vi "Initialize.vi"(8 "error in (no error)":errorcluster, 11 "Core Configuration in":refnum<class "Core Configurations.lvclass">) -> (0 "error out":errorcluster, 3 "Core Configuration out":refnum<class "Core Configurations.lvclass">)   [LabVIEW 2017, in "DSF Core.lvlib" / "Core Configurations.lvclass"]
uses:
  Core Configurations.lvclass
  C:/Git/DSF/Core/Classes/Component Configuration/Component Configurations.lvclass
  Base/Channel/Channel Configuration.lvclass
  C:/Git/DSF/Core/Classes/Configuration/Configuration.lvclass
  Base/Transfer/Transfer Configuration.lvclass
  Base/Group/Group Configuration.lvclass
  Base/Thread/Thread Configuration.lvclass
  Base/Plugin/Plugin Configuration.lvclass
  Component Configuration/Component Configurations.lvclass
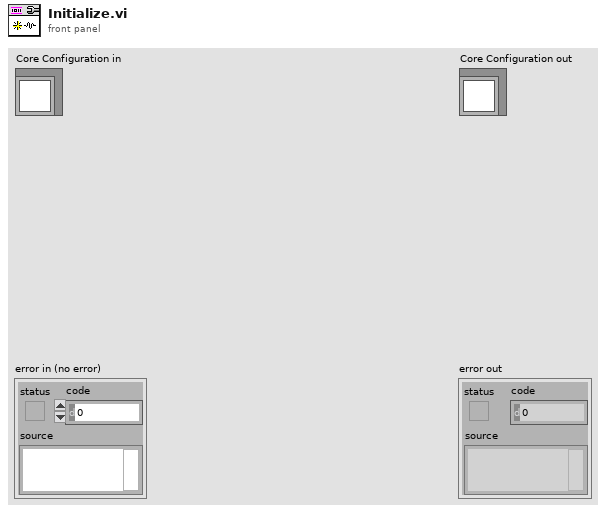
[diagram p1: front panel]
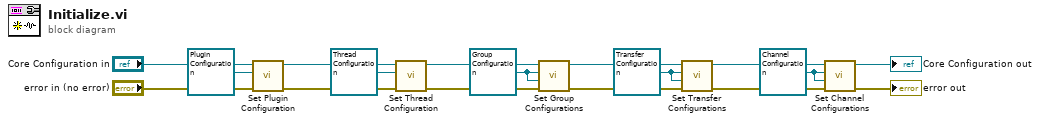
[diagram p0: block diagram]
diagram:
  w3 = refnum<class "Group Configuration.lvclass"> refnum ("DSF Core.lvlib:Group Configuration.lvclass")
  w4 = refnum<class "Transfer Configuration.lvclass"> refnum ("DSF Core.lvlib:Transfer Configuration.lvclass")
  w5 = refnum<class "Channel Configuration.lvclass"> refnum ("DSF Core.lvlib:Core Channel Configuration.lvclass")
  n1 = call "Set Plugin Configuration.vi"("error in (no error)"="error in (no error)", "Plugin Configuration"=refnum<class "Plugin Configuration.lvclass"> refnum ("DSF Core.lvlib:Plugin Configuration.lvclass"), "Component Configuration in"="Core Configuration in") -> ("error out"=w13:errorcluster, "Component Configuration out"=w16:refnum<class "Core Configurations.lvclass">)  [unwired: 7 in]
  n2 = call "Set Thread Configuration.vi"("error in (no error)"=w13, "Thread Configuration"=refnum<class "Thread Configuration.lvclass"> refnum ("DSF Core.lvlib:Thread Configuration.lvclass"), "Component Configuration in"=w16) -> ("error out"=w6:errorcluster, "Component Configuration out"=w15:refnum<class "Core Configurations.lvclass">)  [unwired: 7 in]
  n3 = call "Set Group Configurations.vi"("error in (no error)"=w6, "Tx Group Configuration"=w3, "Rx Group Configuration"=w3, "Component Configuration in"=w15) -> ("error out"=w11:errorcluster, "Component Configuration out"=w12:refnum<class "Core Configurations.lvclass">)  [unwired: 6 in]
  n4 = call "Set Transfer Configurations.vi"("error in (no error)"=w11, "Tx Transfer Configuration"=w4, "Rx Transfer Configuration"=w4, "Component Configuration in"=w12) -> ("error out"=w10:errorcluster, "Component Configuration out"=w9:refnum<class "Core Configurations.lvclass">)  [unwired: 6 in]
  n5 = call "Set Channel Configurations.vi"("error in (no error)"=w10, "Tx Channel Configuration"=w5, "Rx Channel Configuration"=w5, "Component Configuration in"=w9) -> ("error out"=→"error out":errorcluster, "Component Configuration out"=→"Core Configuration out":refnum<class "Core Configurations.lvclass">)  [unwired: 6 in]
